vi "IO Contol.vi"(8 "error in":errorcluster, 11 "IO Operation":T1=enum."Disconnect Digit ALL") -> (0 "error out":errorcluster, 1 "task out":refnum<k21>, 3 "number of samples written per channel":u32)   [LabVIEW 2009]
uses:
  Digit IO control.ctl
  <vilib>/DAQmx/write.llb/DAQmx Write (Digital Bool 1Line 1Point).vi
  <vilib>/DAQmx/write.llb/DAQmx Write (Digital 1D Bool NChan 1Samp 1Line).vi
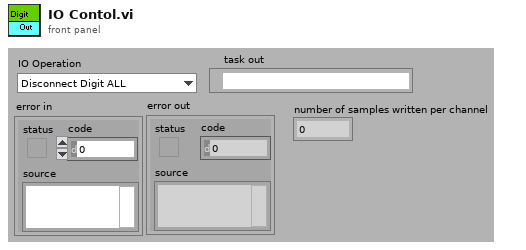
[diagram p1: front panel]
types:
  T1 = typedef "Digit IO control.ctl" = enum16{"Pull X1_4 Low", "Disconnect Pull X1_4 Low", "Down Cylinder", "Disconnect Down Cylinder", "Load X1_1_5", "Disconnect Load X1_1_5", "Measu X1_1_5", "Disconnect Measu X1_1_5", "Measu Z1_1_5", "Disconnect Measu Z1_1_5", "Power X1_1", "Disconnect Power X1_1", "RS232 Power", "Disconnect RS232 Power", "Card Cylinder", "Disconnect Card Cylinder", "Fail LED", "Disconnect Fail LED", "LCA Power", "Disconnect LCA Power", "BeyondCylinderDowndigit", "Disconnect BeyondCylinderDowendigit", "Frequency", "Disconnect Frequency", "Measu Current", "Disconnect Measu Current", "Measu current_1", "Disconnect Measu current_1", "Digit ALL", "Disconnect Digit ALL", "PASS LED", "Disconnect PASS LED", "Load Z1_1_3", "Disconnect Load Z1_1_3", "RS232 Connect", "Disconnect RS232 Connect", "Power Z1_7", "Disconnect Power Z1_7", "Pull Z_1_5  low", "Disconnect Pull Z_1_5  low", "Connect LCA_1", "Disconnect LCA_1", "short LCA", "Disconnect short LCA", "PT100", "Disconnect PT100", "NO connect", "Disconnect NO connect"}
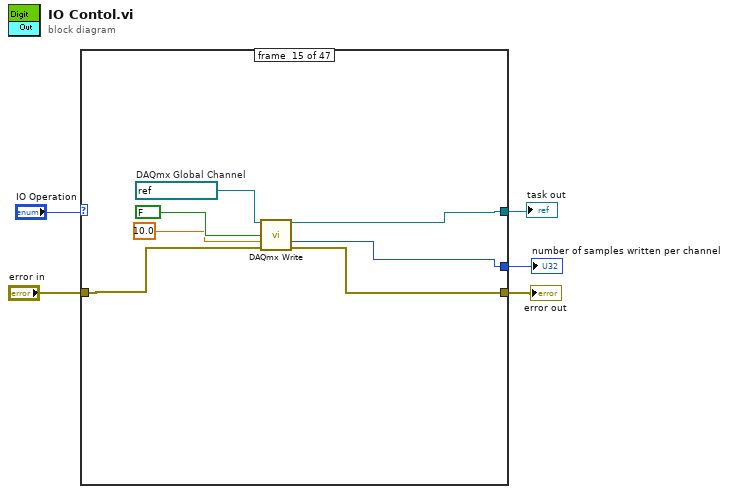
[diagram p0: block diagram]
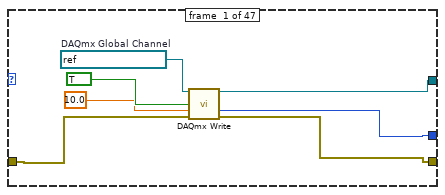
[diagram p2: hidden frame]
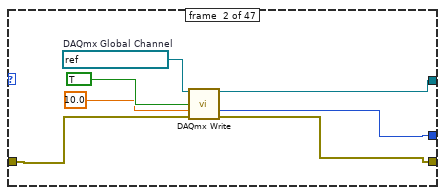
[diagram p3: hidden frame]
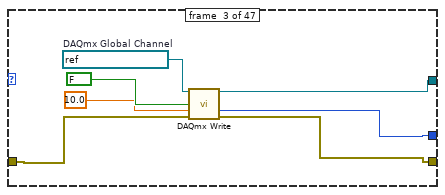
[diagram p4: hidden frame]
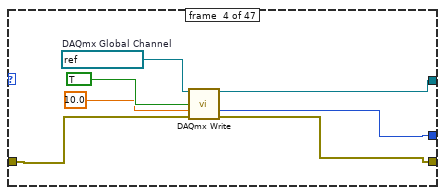
[diagram p5: hidden frame]
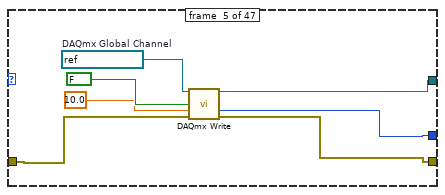
[diagram p6: hidden frame]
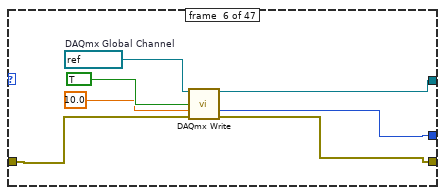
[diagram p7: hidden frame]
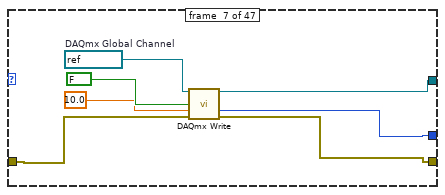
[diagram p8: hidden frame]
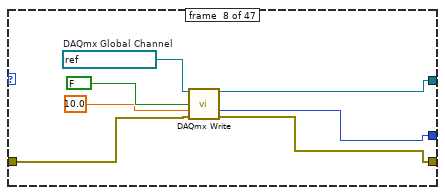
[diagram p9: hidden frame]
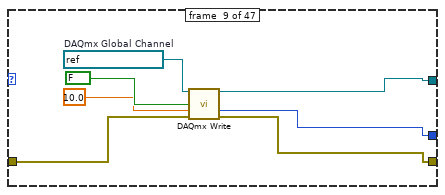
[diagram p10: hidden frame]
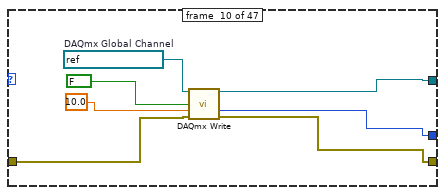
[diagram p11: hidden frame]
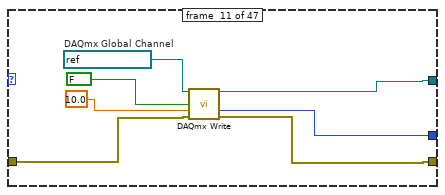
[diagram p12: hidden frame]
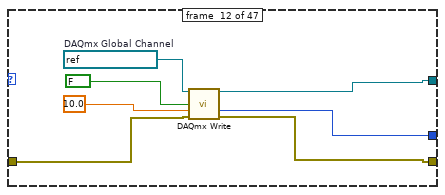
[diagram p13: hidden frame]
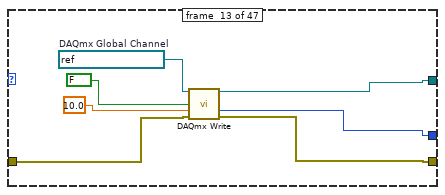
[diagram p14: hidden frame]
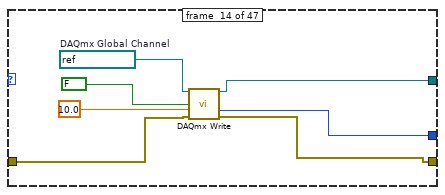
[diagram p15: hidden frame]
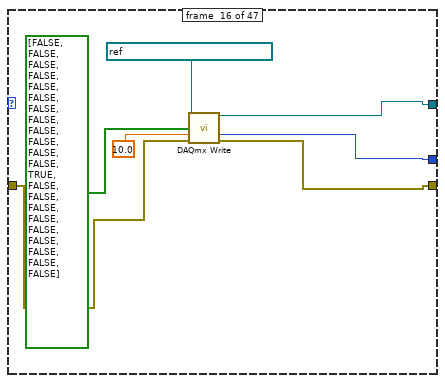
[diagram p16: hidden frame]
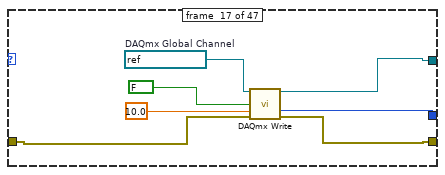
[diagram p17: hidden frame]
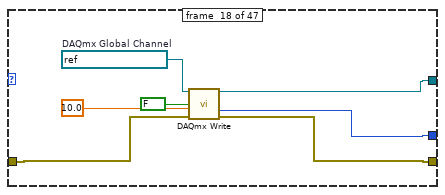
[diagram p18: hidden frame]
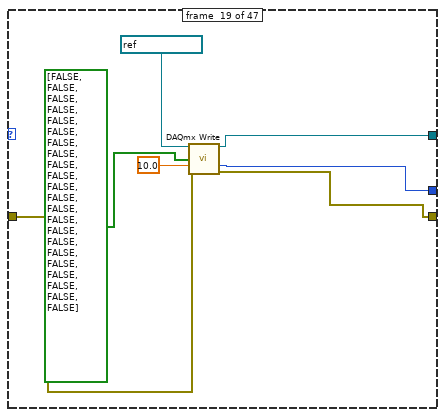
[diagram p19: hidden frame]
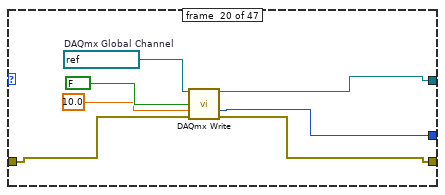
[diagram p20: hidden frame]
diagram:
  n1 = case shown="\"Disconnect short LCA\"" "IO Operation" {
    tunnel: "error in" -> [w10 w17 w24 w31 w38 w45 w52 w59 w66 w73 w80 w87 w94 w101 w107 w115 w122 w128 w136 w142 w150 w157 w163 w171 w178 w185 w191 w197 w205 w212 w219 w226 w233 w240 w247 w254 w261 w268 w275 w282 w289 w296 w304 w310 w317 w324 w331]
    tunnel: [w7 w14 w21 w28 w35 w42 w49 w56 w63 w70 w77 w84 w91 w98 w104 w111 w118 w125 w134 w139 w146 w154 w160 w167 w174 w181 w189 w196 w201 w208 w215 w222 w230 w236 w243 w251 w257 w264 w271 w278 w285 w292 w300 w307 w314 w321 w328] -> w4
    tunnel: [w9 w16 w23 w30 w37 w44 w51 w58 w65 w72 w79 w86 w93 w100 w106 w113 w120 w127 w132 w141 w148 w156 w162 w169 w176 w183 w190 w195 w203 w210 w217 w224 w232 w238 w245 w253 w259 w267 w274 w281 w287 w294 w302 w309 w316 w323 w330] -> w3
    tunnel: [w8 w15 w22 w29 w36 w43 w50 w57 w64 w71 w78 w85 w92 w99 w105 w112 w119 w126 w133 w140 w147 w155 w161 w168 w175 w182 w188 w194 w202 w209 w216 w223 w231 w237 w244 w252 w258 w265 w272 w279 w286 w293 w301 w308 w315 w322 w329] -> w2
    frame #0 {
      w12 = refnum<k21> "Down Cylinder"  # DAQmx Global Channel
      n2 = call-poly <vilib>:"DAQmx Write.vi"("task/channels in"=w12, "data"=TRUE, "timeout"=10.0, "error in"=w10) -> ("task out"=w7:refnum<k21>, "number of samples written per channel"=w8:u32, "error out"=w9:errorcluster)  [unwired: 1 in, 8 out]
    }
    frame #1 {
      w19 = refnum<k21> "Connect LCA_1"  # DAQmx Global Channel
      n3 = call-poly <vilib>:"DAQmx Write.vi"("task/channels in"=w19, "data"=TRUE, "timeout"=10.0, "error in"=w17) -> ("task out"=w14:refnum<k21>, "number of samples written per channel"=w15:u32, "error out"=w16:errorcluster)  [unwired: 1 in, 8 out]
    }
    frame #2 {
      w26 = refnum<k21> "Connect LCA_1"  # DAQmx Global Channel
      n4 = call-poly <vilib>:"DAQmx Write.vi"("task/channels in"=w26, "data"=FALSE, "timeout"=10.0, "error in"=w24) -> ("task out"=w21:refnum<k21>, "number of samples written per channel"=w22:u32, "error out"=w23:errorcluster)  [unwired: 1 in, 8 out]
    }
    frame #3 {
      w33 = refnum<k21> "short LCA"  # DAQmx Global Channel
      n5 = call-poly <vilib>:"DAQmx Write.vi"("task/channels in"=w33, "data"=TRUE, "timeout"=10.0, "error in"=w31) -> ("task out"=w28:refnum<k21>, "number of samples written per channel"=w29:u32, "error out"=w30:errorcluster)  [unwired: 1 in, 8 out]
    }
    frame #4 {
      w40 = refnum<k21> "short LCA"  # DAQmx Global Channel
      n6 = call-poly <vilib>:"DAQmx Write.vi"("task/channels in"=w40, "data"=FALSE, "timeout"=10.0, "error in"=w38) -> ("task out"=w35:refnum<k21>, "number of samples written per channel"=w36:u32, "error out"=w37:errorcluster)  [unwired: 1 in, 8 out]
    }
    frame #5 {
      w47 = refnum<k21> "PT100"  # DAQmx Global Channel
      n7 = call-poly <vilib>:"DAQmx Write.vi"("task/channels in"=w47, "data"=TRUE, "timeout"=10.0, "error in"=w45) -> ("task out"=w42:refnum<k21>, "number of samples written per channel"=w43:u32, "error out"=w44:errorcluster)  [unwired: 1 in, 8 out]
    }
    frame #6 {
      w54 = refnum<k21> "PT100"  # DAQmx Global Channel
      n8 = call-poly <vilib>:"DAQmx Write.vi"("task/channels in"=w54, "data"=FALSE, "timeout"=10.0, "error in"=w52) -> ("task out"=w49:refnum<k21>, "number of samples written per channel"=w50:u32, "error out"=w51:errorcluster)  [unwired: 1 in, 8 out]
    }
    frame #7 {
      w61 = refnum<k21> "Load X1_1_5"  # DAQmx Global Channel
      n9 = call-poly <vilib>:"DAQmx Write.vi"("task/channels in"=w61, "data"=FALSE, "timeout"=10.0, "error in"=w59) -> ("task out"=w56:refnum<k21>, "number of samples written per channel"=w57:u32, "error out"=w58:errorcluster)  [unwired: 1 in, 8 out]
    }
    frame #8 {
      w68 = refnum<k21> "Measu X1_1_5"  # DAQmx Global Channel
      n10 = call-poly <vilib>:"DAQmx Write.vi"("task/channels in"=w68, "data"=FALSE, "timeout"=10.0, "error in"=w66) -> ("task out"=w63:refnum<k21>, "number of samples written per channel"=w64:u32, "error out"=w65:errorcluster)  [unwired: 1 in, 8 out]
    }
    frame #9 {
      w75 = refnum<k21> "Measu Z1_1_5"  # DAQmx Global Channel
      n11 = call-poly <vilib>:"DAQmx Write.vi"("task/channels in"=w75, "data"=FALSE, "timeout"=10.0, "error in"=w73) -> ("task out"=w70:refnum<k21>, "number of samples written per channel"=w71:u32, "error out"=w72:errorcluster)  [unwired: 1 in, 8 out]
    }
    frame #10 {
      w82 = refnum<k21> "Power X1_1"  # DAQmx Global Channel
      n12 = call-poly <vilib>:"DAQmx Write.vi"("task/channels in"=w82, "data"=FALSE, "timeout"=10.0, "error in"=w80) -> ("task out"=w77:refnum<k21>, "number of samples written per channel"=w78:u32, "error out"=w79:errorcluster)  [unwired: 1 in, 8 out]
    }
    frame #11 {
      w89 = refnum<k21> "RS232 Power"  # DAQmx Global Channel
      n13 = call-poly <vilib>:"DAQmx Write.vi"("task/channels in"=w89, "data"=FALSE, "timeout"=10.0, "error in"=w87) -> ("task out"=w84:refnum<k21>, "number of samples written per channel"=w85:u32, "error out"=w86:errorcluster)  [unwired: 1 in, 8 out]
    }
    frame #12 {
      w96 = refnum<k21> "Card Cylinder"  # DAQmx Global Channel
      n14 = call-poly <vilib>:"DAQmx Write.vi"("task/channels in"=w96, "data"=FALSE, "timeout"=10.0, "error in"=w94) -> ("task out"=w91:refnum<k21>, "number of samples written per channel"=w92:u32, "error out"=w93:errorcluster)  [unwired: 1 in, 8 out]
    }
    frame #13 {
      w103 = refnum<k21> "Fail LED"  # DAQmx Global Channel
      n15 = call-poly <vilib>:"DAQmx Write.vi"("task/channels in"=w103, "data"=FALSE, "timeout"=10.0, "error in"=w101) -> ("task out"=w98:refnum<k21>, "number of samples written per channel"=w99:u32, "error out"=w100:errorcluster)  [unwired: 1 in, 8 out]
    }
    frame #14 {
      w110 = refnum<k21> "LCA Power"  # DAQmx Global Channel
      n16 = call-poly <vilib>:"DAQmx Write.vi"("task/channels in"=w110, "data"=FALSE, "timeout"=10.0, "error in"=w107) -> ("task out"=w104:refnum<k21>, "number of samples written per channel"=w105:u32, "error out"=w106:errorcluster)  [unwired: 1 in, 8 out]
    }
    frame #15 {
      n17 = call-poly <vilib>:"DAQmx Write.vi"("task/channels in"=refnum<k21> "BeyondCylinderDowndigit", "data"=bool[] [FALSE, FALSE, FALSE, FALSE, FALSE, FALSE, FALSE, FALSE, FALSE, FALSE, FALSE, FALSE, TRUE, FALSE, FALSE, FALSE, FALSE, FALSE, FALSE, FALSE, FALSE, FALSE], "timeout"=10.0, "error in"=w115) -> ("task out"=w111:refnum<k21>, "number of samples written per channel"=w112:u32, "error out"=w113:errorcluster)  [unwired: 1 in, 8 out]
    }
    frame #16 {
      w124 = refnum<k21> "Frequency"  # DAQmx Global Channel
      n18 = call-poly <vilib>:"DAQmx Write.vi"("task/channels in"=w124, "data"=FALSE, "timeout"=10.0, "error in"=w122) -> ("task out"=w118:refnum<k21>, "number of samples written per channel"=w119:u32, "error out"=w120:errorcluster)  [unwired: 1 in, 8 out]
    }
    frame #17 {
      w131 = refnum<k21> "Measu Current"  # DAQmx Global Channel
      n19 = call-poly <vilib>:"DAQmx Write.vi"("task/channels in"=w131, "data"=FALSE, "timeout"=10.0, "error in"=w128) -> ("task out"=w125:refnum<k21>, "number of samples written per channel"=w126:u32, "error out"=w127:errorcluster)  [unwired: 1 in, 8 out]
    }
    frame #18 {
      n20 = call-poly <vilib>:"DAQmx Write.vi"("task/channels in"=refnum<k21> "Digit ALL", "data"=bool[] [FALSE, FALSE, FALSE, FALSE, FALSE, FALSE, FALSE, FALSE, FALSE, FALSE, FALSE, FALSE, FALSE, FALSE, FALSE, FALSE, FALSE, FALSE, FALSE, FALSE, FALSE, FALSE], "timeout"=10.0, "error in"=w136) -> ("task out"=w134:refnum<k21>, "number of samples written per channel"=w133:u32, "error out"=w132:errorcluster)  [unwired: 1 in, 8 out]
    }
    frame #19 {
      w145 = refnum<k21> "PASS LED"  # DAQmx Global Channel
      n21 = call-poly <vilib>:"DAQmx Write.vi"("task/channels in"=w145, "data"=FALSE, "timeout"=10.0, "error in"=w142) -> ("task out"=w139:refnum<k21>, "number of samples written per channel"=w140:u32, "error out"=w141:errorcluster)  [unwired: 1 in, 8 out]
    }
    frame #20 {
      w152 = refnum<k21> "Load Z1_1_3"  # DAQmx Global Channel
      n22 = call-poly <vilib>:"DAQmx Write.vi"("task/channels in"=w152, "data"=FALSE, "timeout"=10.0, "error in"=w150) -> ("task out"=w146:refnum<k21>, "number of samples written per channel"=w147:u32, "error out"=w148:errorcluster)  [unwired: 1 in, 8 out]
    }
    frame #21 {
      w159 = refnum<k21> "RS232 Connect"  # DAQmx Global Channel
      n23 = call-poly <vilib>:"DAQmx Write.vi"("task/channels in"=w159, "data"=FALSE, "timeout"=10.0, "error in"=w157) -> ("task out"=w154:refnum<k21>, "number of samples written per channel"=w155:u32, "error out"=w156:errorcluster)  [unwired: 1 in, 8 out]
    }
    frame #22 {
      w166 = refnum<k21> "Power Z1_7"  # DAQmx Global Channel
      n24 = call-poly <vilib>:"DAQmx Write.vi"("task/channels in"=w166, "data"=FALSE, "timeout"=10.0, "error in"=w163) -> ("task out"=w160:refnum<k21>, "number of samples written per channel"=w161:u32, "error out"=w162:errorcluster)  [unwired: 1 in, 8 out]
    }
    frame #23 {
      w173 = refnum<k21> "Pull X1_4 Low"  # DAQmx Global Channel
      n25 = call-poly <vilib>:"DAQmx Write.vi"("task/channels in"=w173, "data"=FALSE, "timeout"=10.0, "error in"=w171) -> ("task out"=w167:refnum<k21>, "number of samples written per channel"=w168:u32, "error out"=w169:errorcluster)  [unwired: 1 in, 8 out]
    }
    frame #24 {
      w180 = refnum<k21> "Pull Z1_5 low"  # DAQmx Global Channel
      n26 = call-poly <vilib>:"DAQmx Write.vi"("task/channels in"=w180, "data"=FALSE, "timeout"=10.0, "error in"=w178) -> ("task out"=w174:refnum<k21>, "number of samples written per channel"=w175:u32, "error out"=w176:errorcluster)  [unwired: 1 in, 8 out]
    }
    frame #25 {
      w187 = refnum<k21> "LCA Power"  # DAQmx Global Channel
      n27 = call-poly <vilib>:"DAQmx Write.vi"("task/channels in"=w187, "data"=TRUE, "timeout"=10.0, "error in"=w185) -> ("task out"=w181:refnum<k21>, "number of samples written per channel"=w182:u32, "error out"=w183:errorcluster)  [unwired: 1 in, 8 out]
    }
    frame #26 {
      w193 = refnum<k21> "Pull X1_4 Low"  # DAQmx Global Channel
      n28 = call-poly <vilib>:"DAQmx Write.vi"("task/channels in"=w193, "data"=TRUE, "error in"=w191) -> ("task out"=w189:refnum<k21>, "number of samples written per channel"=w188:u32, "error out"=w190:errorcluster)  [unwired: 1 in, 9 out]
    }
    frame #27 {
      w200 = refnum<k21> "Down Cylinder"  # DAQmx Global Channel
      n29 = call-poly <vilib>:"DAQmx Write.vi"("task/channels in"=w200, "data"=FALSE, "timeout"=10.0, "error in"=w197) -> ("task out"=w196:refnum<k21>, "number of samples written per channel"=w194:u32, "error out"=w195:errorcluster)  [unwired: 1 in, 8 out]
    }
    frame #28 {
      w207 = refnum<k21> "Load X1_1_5"  # DAQmx Global Channel
      n30 = call-poly <vilib>:"DAQmx Write.vi"("task/channels in"=w207, "data"=TRUE, "timeout"=10.0, "error in"=w205) -> ("task out"=w201:refnum<k21>, "number of samples written per channel"=w202:u32, "error out"=w203:errorcluster)  [unwired: 1 in, 8 out]
    }
    frame #29 {
      w214 = refnum<k21> "Measu X1_1_5"  # DAQmx Global Channel
      n31 = call-poly <vilib>:"DAQmx Write.vi"("task/channels in"=w214, "data"=TRUE, "timeout"=10.0, "error in"=w212) -> ("task out"=w208:refnum<k21>, "number of samples written per channel"=w209:u32, "error out"=w210:errorcluster)  [unwired: 1 in, 8 out]
    }
    frame #30 {
      w221 = refnum<k21> "Measu Z1_1_5"  # DAQmx Global Channel
      n32 = call-poly <vilib>:"DAQmx Write.vi"("task/channels in"=w221, "data"=TRUE, "timeout"=10.0, "error in"=w219) -> ("task out"=w215:refnum<k21>, "number of samples written per channel"=w216:u32, "error out"=w217:errorcluster)  [unwired: 1 in, 8 out]
    }
    frame #31 {
      w228 = refnum<k21> "Power X1_1"  # DAQmx Global Channel
      n33 = call-poly <vilib>:"DAQmx Write.vi"("task/channels in"=w228, "data"=TRUE, "timeout"=10.0, "error in"=w226) -> ("task out"=w222:refnum<k21>, "number of samples written per channel"=w223:u32, "error out"=w224:errorcluster)  [unwired: 1 in, 8 out]
    }
    frame #32 {
      w235 = refnum<k21> "RS232 Power"  # DAQmx Global Channel
      n34 = call-poly <vilib>:"DAQmx Write.vi"("task/channels in"=w235, "data"=TRUE, "timeout"=10.0, "error in"=w233) -> ("task out"=w230:refnum<k21>, "number of samples written per channel"=w231:u32, "error out"=w232:errorcluster)  [unwired: 1 in, 8 out]
    }
    frame #33 {
      w242 = refnum<k21> "Card Cylinder"  # DAQmx Global Channel
      n35 = call-poly <vilib>:"DAQmx Write.vi"("task/channels in"=w242, "data"=TRUE, "timeout"=10.0, "error in"=w240) -> ("task out"=w236:refnum<k21>, "number of samples written per channel"=w237:u32, "error out"=w238:errorcluster)  [unwired: 1 in, 8 out]
    }
    frame #34 {
      w249 = refnum<k21> "Fail LED"  # DAQmx Global Channel
      n36 = call-poly <vilib>:"DAQmx Write.vi"("task/channels in"=w249, "data"=TRUE, "timeout"=10.0, "error in"=w247) -> ("task out"=w243:refnum<k21>, "number of samples written per channel"=w244:u32, "error out"=w245:errorcluster)  [unwired: 1 in, 8 out]
    }
    frame #35 {
      n37 = call-poly <vilib>:"DAQmx Write.vi"("task/channels in"=refnum<k21> "BeyondCylinderDowndigit", "data"=bool[] [FALSE, FALSE, FALSE, FALSE, FALSE, FALSE, FALSE, FALSE, FALSE, FALSE, FALSE, FALSE, TRUE, FALSE, FALSE, FALSE, FALSE, FALSE, FALSE, FALSE, FALSE, FALSE], "timeout"=10.0, "error in"=w254) -> ("task out"=w251:refnum<k21>, "number of samples written per channel"=w252:u32, "error out"=w253:errorcluster)  [unwired: 1 in, 8 out]
    }
    frame #36 {
      w263 = refnum<k21> "Frequency"  # DAQmx Global Channel
      n38 = call-poly <vilib>:"DAQmx Write.vi"("task/channels in"=w263, "data"=TRUE, "timeout"=10.0, "error in"=w261) -> ("task out"=w257:refnum<k21>, "number of samples written per channel"=w258:u32, "error out"=w259:errorcluster)  [unwired: 1 in, 8 out]
    }
    frame #37 {
      w270 = refnum<k21> "Measu Current"  # DAQmx Global Channel
      n39 = call-poly <vilib>:"DAQmx Write.vi"("task/channels in"=w270, "data"=TRUE, "timeout"=10.0, "error in"=w268) -> ("task out"=w264:refnum<k21>, "number of samples written per channel"=w265:u32, "error out"=w267:errorcluster)  [unwired: 1 in, 8 out]
    }
    frame #38 {
      w277 = refnum<k21> "Measu Current_1"  # DAQmx Global Channel
      n40 = call-poly <vilib>:"DAQmx Write.vi"("task/channels in"=w277, "data"=TRUE, "timeout"=10.0, "error in"=w275) -> ("task out"=w271:refnum<k21>, "number of samples written per channel"=w272:u32, "error out"=w274:errorcluster)  [unwired: 1 in, 8 out]
    }
    frame #39 {
      w284 = refnum<k21> "Measu Current_1"  # DAQmx Global Channel
      n41 = call-poly <vilib>:"DAQmx Write.vi"("task/channels in"=w284, "data"=FALSE, "timeout"=10.0, "error in"=w282) -> ("task out"=w278:refnum<k21>, "number of samples written per channel"=w279:u32, "error out"=w281:errorcluster)  [unwired: 1 in, 8 out]
    }
    frame #40 {
      w291 = refnum<k21> "Load Z1_1_3"  # DAQmx Global Channel
      n42 = call-poly <vilib>:"DAQmx Write.vi"("task/channels in"=w291, "data"=TRUE, "timeout"=10.0, "error in"=w289) -> ("task out"=w285:refnum<k21>, "number of samples written per channel"=w286:u32, "error out"=w287:errorcluster)  [unwired: 1 in, 8 out]
    }
    frame #41 {
      w298 = refnum<k21> "PASS LED"  # DAQmx Global Channel
      n43 = call-poly <vilib>:"DAQmx Write.vi"("task/channels in"=w298, "data"=TRUE, "timeout"=10.0, "error in"=w296) -> ("task out"=w292:refnum<k21>, "number of samples written per channel"=w293:u32, "error out"=w294:errorcluster)  [unwired: 1 in, 8 out]
    }
    frame #42 {
      n44 = call-poly <vilib>:"DAQmx Write.vi"("task/channels in"=refnum<k21> "Digit ALL", "data"=bool[] [FALSE, FALSE, FALSE, FALSE, FALSE, FALSE, FALSE, FALSE, FALSE, FALSE, FALSE, FALSE, FALSE, FALSE, FALSE, FALSE, FALSE, FALSE, FALSE, FALSE, FALSE, FALSE], "timeout"=10.0, "error in"=w304) -> ("task out"=w300:refnum<k21>, "number of samples written per channel"=w301:u32, "error out"=w302:errorcluster)  [unwired: 1 in, 8 out]
    }
    frame #43 {
      w312 = refnum<k21> "RS232 Connect"  # DAQmx Global Channel
      n45 = call-poly <vilib>:"DAQmx Write.vi"("task/channels in"=w312, "data"=TRUE, "timeout"=10.0, "error in"=w310) -> ("task out"=w307:refnum<k21>, "number of samples written per channel"=w308:u32, "error out"=w309:errorcluster)  [unwired: 1 in, 8 out]
    }
    frame #44 {
      w319 = refnum<k21> "Power Z1_7"  # DAQmx Global Channel
      n46 = call-poly <vilib>:"DAQmx Write.vi"("task/channels in"=w319, "data"=TRUE, "timeout"=10.0, "error in"=w317) -> ("task out"=w314:refnum<k21>, "number of samples written per channel"=w315:u32, "error out"=w316:errorcluster)  [unwired: 1 in, 8 out]
    }
    frame #45 {
      w326 = refnum<k21> "Pull Z1_5 low"  # DAQmx Global Channel
      n47 = call-poly <vilib>:"DAQmx Write.vi"("task/channels in"=w326, "data"=TRUE, "timeout"=10.0, "error in"=w324) -> ("task out"=w321:refnum<k21>, "number of samples written per channel"=w322:u32, "error out"=w323:errorcluster)  [unwired: 1 in, 8 out]
    }
    frame #46 {
      w333 = refnum<k21> "NO connect"  # DAQmx Global Channel
      n48 = call-poly <vilib>:"DAQmx Write.vi"("task/channels in"=w333, "data"=TRUE, "timeout"=10.0, "error in"=w331) -> ("task out"=w328:refnum<k21>, "number of samples written per channel"=w329:u32, "error out"=w330:errorcluster)  [unwired: 1 in, 8 out]
    }
  }
  "error out" <- w3
  "number of samples written per channel" <- w2
  "task out" <- w4
